vi "Handle Timeout.vi"(8 "error in (no error)":errorcluster, 11 "Transfer Line in":refnum<class "Transfer Line.lvclass">) -> (0 "error out":errorcluster, 3 "Transfer Line out":refnum<class "Transfer Line.lvclass">)   [LabVIEW 2015, in "cRIO-Carbondioxide.lvlib" / "CO2-Actor.lvlib" / "Transfer Line.lvclass"]
uses:
  Transfer Line.lvclass
  Transfer Line.lvclass/Transfer Line.ctl
  <vilib>/ActorFramework/Actor/Actor.lvclass/Actor.ctl
  <vilib>/ActorFramework/Message Enqueuer/Message Enqueuer.lvclass/Message Enqueuer.ctl
  Controls/Vacuum State Enumerator.ctl
  <vilib>/ActorFramework/Message Enqueuer/Message Priority.ctl
  subs/Sample/Sample.lvclass/Sample.ctl
  Transfer Line Messages/Sample In Msg/Sample In Msg.lvclass/Sample In Msg.ctl
  <vilib>/ActorFramework/Actor/Read Self Enqueuer.vi
  <vilib>/ActorFramework/Message Enqueuer/Enqueue.vi
  <vilib>/ActorFramework/Message Enqueuer/Init from Existing Queue.vi
  <vilib>/ActorFramework/Message Priority Queue/Priority Enqueue.vi
  subs/Sample/Read Sample From Container.vi
  <vilib>/ActorFramework/Actor/Actor.lvclass
  <vilib>/ActorFramework/Message Enqueuer/Message Enqueuer.lvclass
  Transfer Line Messages/Sample Out Msg/Sample Out Msg.lvclass
  Transfer Line Messages/Sample In Msg/Sample In Msg.lvclass
  subs/Sample/Sample.lvclass
  CO2 Actor/CO2 Actor.lvclass
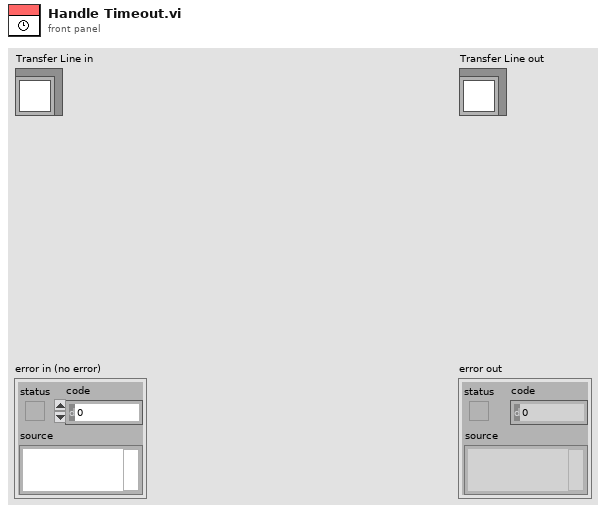
[diagram p1: front panel]
types:
  T1 = typedef "Vacuum State Enumerator.ctl" = enum16{"Pressure Rising", "Plateau", "Pressure Dropping", "Valley", "Low Valley", "Leak", "Unknown"}
  T2 = typedef "Actor Framework.lvlib/Message Enqueuer.lvclass/Message Priority.ctl" = enum16{"Low", "Normal", "High"}
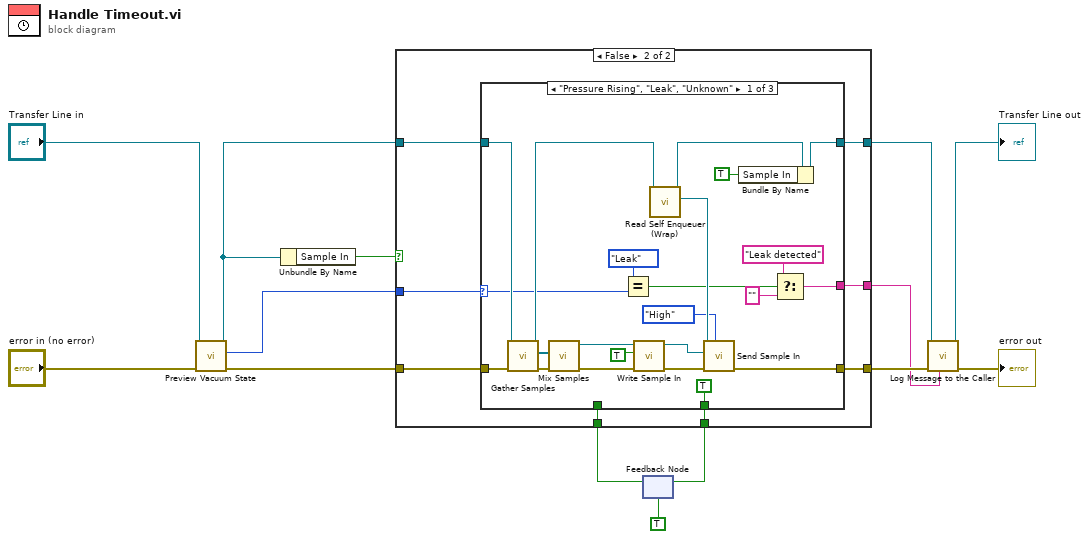
[diagram p0: block diagram]
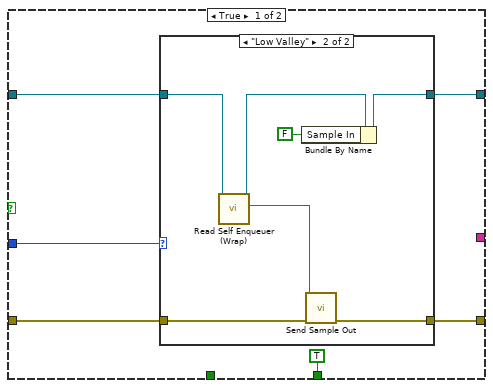
[diagram p2: hidden frame]
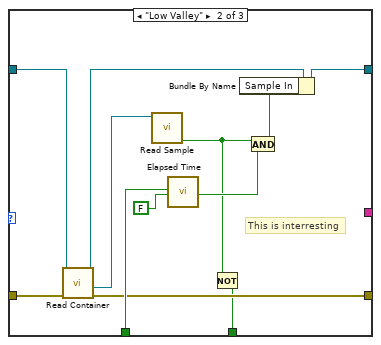
[diagram p4: hidden frame]
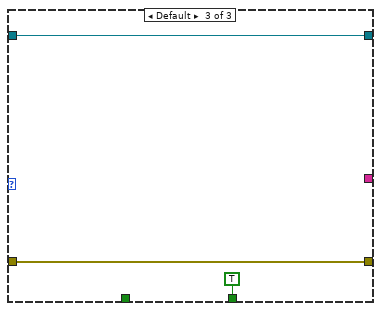
[diagram p5: hidden frame]
diagram:
  n1 = call "Preview Vacuum State.vi"("error in (no error)"="error in (no error)", "Transfer Line in"="Transfer Line in") -> ("error out"=w11:errorcluster, "Vacuum State"=w12:T1, "Transfer Line out"=w10:refnum<class "Transfer Line.lvclass">)  [unwired: 7 in]
  n2 = Unbundle By Name(w10) -> ("Sample In"=w9:bool)
  n3 = feedback #1(TRUE) -> (w7:bool)
  n4 = case shown="False" w9 {
    tunnel: w10 -> [w18 w35]
    tunnel: [w17 w34] -> w3
    tunnel: w11 -> [w20 w37]
    tunnel: [w19 w36] -> w5
    tunnel: w12 -> [w16 w33]
    tunnel: w7 -> [_ w32]
    tunnel: [TRUE w31] -> w6
    tunnel: [_ w30] -> w1
    frame True {
      n5 = case shown="\"Low Valley\"" w16 {
        tunnel: w20 -> [w22 w29]
        tunnel: [w22 w28] -> w19
        tunnel: w18 -> [w21 w26]
        tunnel: [w21 w24] -> w17
        frame "Unknown", Default {
        }
        frame "Low Valley" {
          n6 = call "Read Self Enqueuer (Wrap).vi"("CO2 Actor in"=w26) -> ("Actor Framework:Message Enqueuer"=w27:refnum<class "Message Enqueuer.lvclass">, "CO2 Actor out"=w25:refnum<class "Transfer Line.lvclass">)  [unwired: 9 in]
          n7 = Bundle By Name(cluster=w25, "Sample In"=FALSE) -> (w24:refnum<class "Transfer Line.lvclass">)
          n8 = call "Send Sample Out.vi"("error in (no error)"=w29, "Message Enqueuer"=w27) -> ("error out"=w28:errorcluster)  [unwired: 8 in, 1 out]
        }
      }
    }
    frame False {
      n9 = case shown="\"Pressure Rising\", \"Leak\", \"Unknown\"" w33 {
        selector: w33 -> [w44 _ _]
        tunnel: w37 -> [w57 w69 w75]
        tunnel: [w60 w68 w75] -> w36
        tunnel: w35 -> [w56 w67 w74]
        tunnel: [w47 w70 w74] -> w34
        tunnel: w32 -> [_ w72 _]
        tunnel: [TRUE w61 TRUE] -> w31
        tunnel: [w39 _ _] -> w30
        frame "Pressure Rising", "Leak", "Unknown" {
          n10 = call "Gather Samples.vi"("error in (no error)"=w57, "Transfer Line in"=w56) -> ("error out"=w54:errorcluster, "Samples"=w53:refnum<class "Sample.lvclass">[], "Transfer Line out"=w55:refnum<class "Transfer Line.lvclass">)  [unwired: 7 in]
          n11 = call "Mix Samples.vi"("error in (no error)"=w54, "Samples In"=w53) -> ("error out"=w52:errorcluster, "Sample out"=w49:refnum<class "Sample.lvclass">)  [unwired: 6 in, 2 out]
          n12 = Equal?(x=Vacuum_State_Enumerator."Leak" ("Vacuum State"), y=w44) -> (x = y?=w42:bool)
          n13 = call "Write Sample In.vi"("error in (no error)"=w52, "Sample In"=TRUE, "Sample in"=w49) -> ("error out"=w50:errorcluster, "Sample out"=w51:refnum<class "Sample.lvclass">)  [unwired: 7 in]
          n14 = call "Read Self Enqueuer (Wrap).vi"("CO2 Actor in"=w55) -> ("Actor Framework:Message Enqueuer"=w59:refnum<class "Message Enqueuer.lvclass">, "CO2 Actor out"=w58:refnum<class "Transfer Line.lvclass">)  [unwired: 9 in]
          n15 = call "Send Sample In.vi"("Message Priority (Normal)"=Message_Priority."High", "error in (no error)"=w50, "Sample"=w51, "Message Enqueuer"=w59) -> ("error out"=w60:errorcluster)  [unwired: 6 in, 1 out]
          n16 = Bundle By Name(cluster=w58, "Sample In"=TRUE) -> (w47:refnum<class "Transfer Line.lvclass">)
          n17 = Select(t="Leak detected", s=w42, f="") -> (s? t:f=w39:string)
        }
        frame "Low Valley" {
          # "This is interresting"
          n18 = call "Read Container.vi"("error in (no error)"=w69, "Transfer Line in"=w67) -> ("error out"=w68:errorcluster, "Sample"=w65:refnum<class "Sample.lvclass">, "Transfer Line out"=w66:refnum<class "Transfer Line.lvclass">)  [unwired: 5 in, 2 out]
          n19 = call "Read Sample.vi"("Sample in"=w65) -> ("Sample In"=w62:bool)  [unwired: 6 in, 4 out]
          n20 = call "Elapsed Time"("Reset"=w72, "Auto Reset"=FALSE) -> ("Time has Elapsed"=w64:bool)  [unwired: 10 in, 7 out]
          n21 = Not(x=w62) -> (.not. x?=w61:bool)
          n22 = And(x=w62, y=w64) -> (x .and. y?=w63:bool)
          n23 = Bundle By Name(cluster=w66, "Sample In"=w63) -> (w70:refnum<class "Transfer Line.lvclass">)
        }
        frame Default {
        }
      }
    }
  }
  n24 = feedback-in #1(w6) -> ()
  n25 = call-dynamic "Log Message to the Caller.vi"("String (\"\" = no message to send)"=w1, "error in (no error)"=w5, "CO2 Actor in"=w3) -> ("error out"=→"error out":errorcluster, "CO2 Actor out"=→"Transfer Line out":refnum<class "Transfer Line.lvclass">)  [unwired: 7 in]
